vi "Get Channels.vi"(8 "error in (no error)":errorcluster, 11 "Channel Group in":refnum<k20>) -> (0 "error out":errorcluster, 2 "Channels":refnum<k20>[](array[refnum]), 3 "Channel Group out":refnum<k20>)   [LabVIEW 2015, in "Engine Simulation Toolkit System Explorer.lvlib" / "File Interface.lvlib"]
uses:
  File Interface.lvlib
  <vilib>/Platform/storage/Storage.llb/Get Property (Storage Refnums).vi
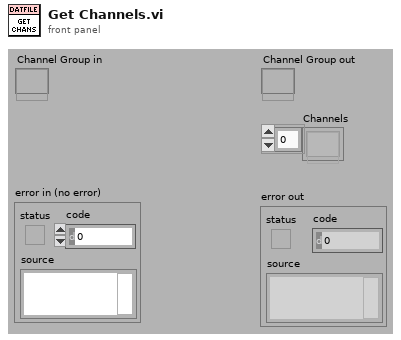
[diagram p1: front panel]
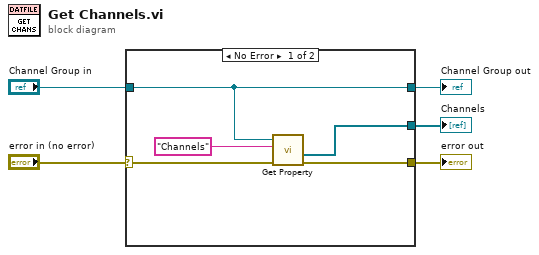
[diagram p0: block diagram]
diagram:
  n1 = case shown="No Error" "error in (no error)" {
    selector: "error in (no error)" -> [w9 w12]
    tunnel: [w6 w12] -> w5
    tunnel: [w8 w11] -> w3
    tunnel: "Channel Group in" -> [w8 w11]
    tunnel: [w7 _] -> w1
    frame No Error {
      n2 = call-poly <vilib>:"Get Property.vi"("error in (no error)"=w9, "Property name"="Channels" ("PropertyName"), "storage refnum"=w8) -> ("error out"=w6:errorcluster, "Value"=w7:refnum<k20>[])  [unwired: 7 out]
    }
    frame Error {
    }
  }
  "Channel Group out" <- w3
  "error out" <- w5
  "Channels" <- w1
